vi "gui_formatData.vi"(7 "ykgw":dbl[](array[numeric]), 8 "error in (no error)":errorcluster, 9 "row size":i32, 10 "Modbus Data":T2, 11 "Data in":string[][](array[string])) -> (0 "error out":errorcluster, 2 "report data":string[](array[string]), 3 "Data out":string[][](array[string]), 4 "SHOWN DATA":T1)   [LabVIEW 2019]
uses:
  instrument/instr_dataCluster.ctl
  core/core shown data.ctl
  instrument/Instrument.lvclass
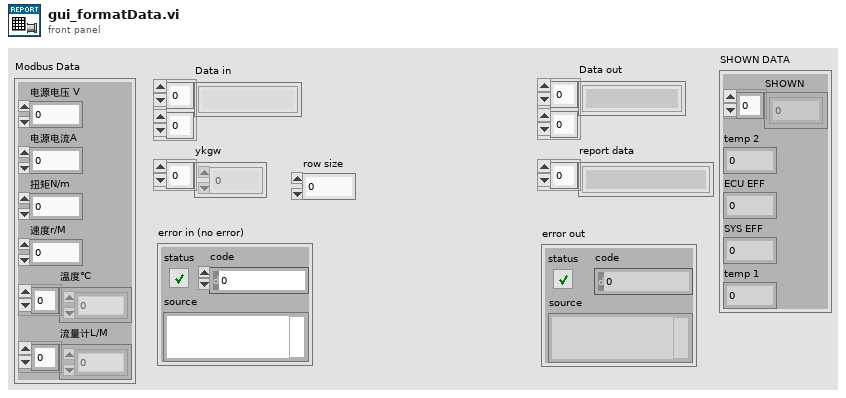
[diagram p1: front panel]
types:
  T1 = typedef "core shown data.ctl" = cluster{"SHOWN":dbl[], "temp 2":dbl, "ECU EFF":dbl, "SYS EFF":dbl, "temp 1":dbl}
  T2 = typedef "Instrument.lvclass/instr_dataCluster.ctl" = cluster{"电源电压 V":dbl, "电源电流A":dbl, "扭矩N/m":dbl, "速度r/M":dbl, "温度℃":dbl[], "流量计L/M":dbl[]}
  T3 = typedef "ecu_dataCluster.ctl" = cluster{"MCU_MotCtrlrSts":dbl, "MCU_MotTq":dbl, "MCU_MotBusU":dbl, "MCU_MotSpd":dbl, "MCU_MotBodyT":dbl, "MCU_MotBody_T":dbl, "MCU_MotCtrlrT":dbl, "MCU 状态":bool, "ErrMsg":i64}
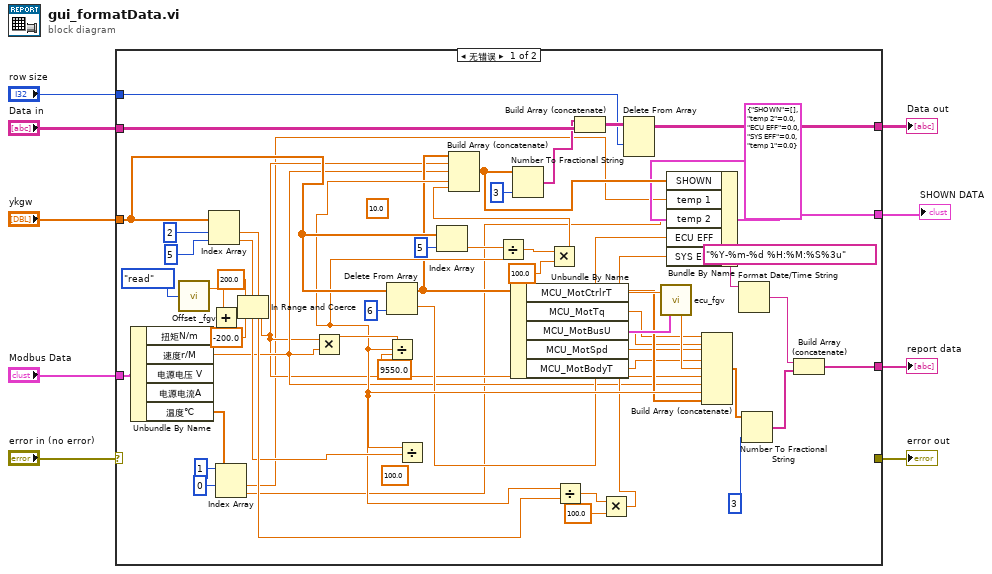
[diagram p0: block diagram]
diagram:
  n1 = case shown="无错误" "error in (no error)" {
    selector: "error in (no error)" -> [_ w64]
    tunnel: "Modbus Data" -> [w63 _]
    tunnel: "ykgw" -> [w35 _]
    tunnel: "Data in" -> [w60 _]
    tunnel: [w58 _] -> w6
    tunnel: "row size" -> [w57 _]
    tunnel: [_ w64] -> w3
    tunnel: [w52 _] -> w2
    tunnel: [w29 _] -> w1
    frame No Error {
      (unwired) 100.0 ("y")
      (unwired) 10.0 ("y")
      n2 = Unbundle By Name(w63) -> ("扭矩N/m"=w23:dbl, "速度r/M"=w26:dbl, "温度℃"=w14:dbl[])  [unwired: 2 out]
      n3 = call "Offset _fgv.vi"("mode"=enum16{"read", "write"}."read") -> ("Value out"=w24:dbl)  [unwired: 2 in, 1 out]
      n4 = Index Array(array=w35, index #1=2 ("index"), index #2=5 ("index")) -> (element #1=w38:dbl, element #2=w36:dbl)
      n5 = Add(x=w24, y=w23) -> (x+y=w21:dbl)
      n6 = Index Array(array=w14, index #1=0 ("索引"), index #2=1 ("索引")) -> (element #1=w11:dbl, element #2=w10:dbl)
      n7 = In Range and Coerce(upper limit=200.0 ("上限"), x=w21, lower limit=-200.0 ("下限")) -> (coerced(x)=w22:dbl)  [unwired: 1 out]
      n8 = Multiply(x=w22, y=w26) -> (x*y=w46:dbl)
      n9 = Delete From Array(array=w35, index=6) -> (deleted portion=w32:dbl, array with subset deleted=w27:dbl[])  [unwired: 1 in]
      n10 = Divide(x=w46, y=9550.0) -> (x/y=w34:dbl)
      n11 = Divide(x=w34, y=w36) -> ()  [unwired: 1 out]
      n12 = Index Array(array=w35, index=5 ("索引")) -> (element=w44:dbl)
      n13 = Divide(x=w34, y=w44) -> (x/y=w42:dbl)
      n14 = Multiply(x=w42, y=100.0) -> (x*y=w41:dbl)
      n15 = Build Array (concatenate)(w27, w22, w26, w34, w41) -> (w33:dbl[])
      n16 = Number To Fractional String(number=w33, precision (6)=i16 3) -> (F-format string=w28:string[])  [unwired: 2 in]
      n17 = Divide(x=w34, y=w38) -> (x/y=w39:dbl)
      n18 = Build Array (concatenate)(w28, w60) -> (w59:string[][])
      n19 = Multiply(x=w39, y=100.0) -> (x*y=w31:dbl)
      n20 = Delete From Array(array=w59, index (row)=w57) -> (array with subset deleted=w58:string[][])  [unwired: 2 in, 1 out]
      n21 = call "ecu_fgv.vi"() -> ("data out"=w49:T3)  [unwired: 10 in, 1 out]
      n22 = Unbundle By Name(w49) -> ("MCU_MotCtrlrT"=w48:dbl, "MCU_MotTq"=w18:dbl, "MCU_MotBusU"=w17:dbl, "MCU_MotSpd"=w16:dbl, "MCU_MotBodyT"=w15:dbl)
      n23 = Bundle By Name(cluster=T1 {"SHOWN"=[], "temp 2"=0.0, "ECU EFF"=0.0, "SYS EFF"=0.0, "temp 1"=0.0} ("SHOWN DATA"), "SHOWN"=w33, "temp 1"=w11, "temp 2"=w10, "ECU EFF"=w32, "SYS EFF"=w31) -> (w29:T1)
      n24 = Build Array (concatenate)(w18, w17, w16, w15, w48, w22, w26, w34, w27) -> (w56:dbl[])
      n25 = Format Date/Time String(time format string (%c)="%Y-%m-%d %H:%M:%S%3u") -> (date/time string=w51:string)  [unwired: 2 in]
      n26 = Number To Fractional String(number=w56, precision (6)=i16 3 ("精度(6)")) -> (F-format string=w55:string[])  [unwired: 2 in]
      n27 = Build Array (concatenate)(w51, w55) -> (w52:string[])
    }
    frame Error {
    }
  }
  "Data out" <- w6
  "error out" <- w3
  "report data" <- w2
  "SHOWN DATA" <- w1
